vi "RSZVB Read Long Data.vi"(8 "error in (no error)":errorcluster {"code" format="%.0x"}, 11 "VISA resource name":refnum<visa-resource-name>) -> (0 "error out":errorcluster {"code" format="%.0x"}, 2 "Data":string, 3 "VISA resource name out":refnum<visa-resource-name>)   [LabVIEW 2011]
doc: "This VI reads a long data from instrument, when length of data is unknown."
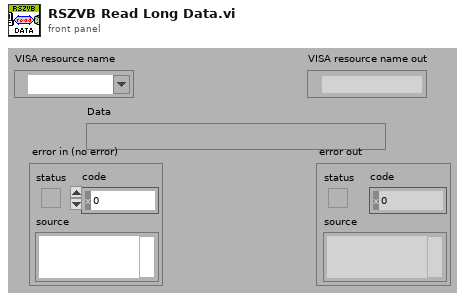
[diagram p1: front panel]
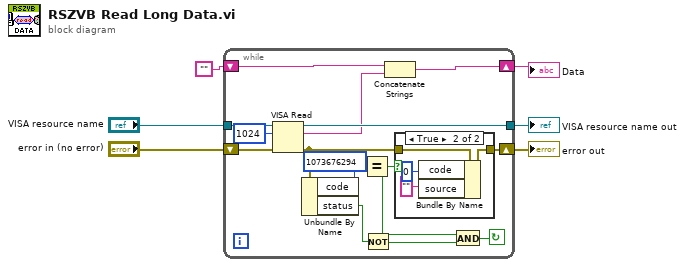
[diagram p0: block diagram]
diagram:
  n1 = while {
    shift-left: "error in (no error)" -> [w16]
    shift-right: [w9] -> w1
    shift-left: "" -> [w17]
    shift-right: [w18] -> w3
    tunnel: "VISA resource name" -> [w20]
    tunnel: [w21] -> w5
    stop <- w15 continue-if-true
    n2 = VISA Read(VISA resource name=w20, byte count=u32 1024 ("byte count (0)"), error in (no error)=w16) -> (VISA resource name out=w21:refnum<visa-resource-name>, read buffer=w19:string, error out=w10:errorcluster)  [unwired: 1 out]
    n3 = Unbundle By Name(w10) -> ("code"=w12:i32, "status"=w13:bool)
    n4 = Equal?(x=1073676294, y=w12) -> (x = y?=w7:bool)
    n5 = Not(x=w13) -> (.not. x?=w8:bool)
    n6 = Concatenate Strings(w17, w19) -> (w18:string)
    n7 = case shown="True" w7 {
      tunnel: w10 -> [w22 w24]
      tunnel: [w22 w23] -> w9
      frame False {
      }
      frame True {
        n8 = Bundle By Name(cluster=w24, "code"=0, "source"="") -> (w23:errorcluster)
      }
    }
    n9 = And(x=w7, y=w8) -> (x .and. y?=w15:bool)
  }
  "Data" <- w3
  "VISA resource name out" <- w5
  "error out" <- w1
